vi "USRP Packet Receiver_Global.vi"() -> ()   [LabVIEW 2013]
uses:
  Global 1.vi
  <vilib>/addons/Modulation/niDMT.lvlib
panel:
  in  "16-PSK System Parameters":T1={"Samples per Symbol"=8, "symbol map"=[], "Differential PSK"=enum."disable", "PSK type"=0} {"PSK type" items=["normal", "shifted", "offset"]; "symbol map" format="%.3f"}
  in  "8-PSK System Parameters":T1={"Samples per Symbol"=8, "symbol map"=[], "Differential PSK"=enum."disable", "PSK type"=0} {"PSK type" items=["normal", "shifted", "offset"]; "symbol map" format="%.3f"}
  in  "QPSK System Parameters":T1={"Samples per Symbol"=8, "symbol map"=[], "Differential PSK"=enum."disable", "PSK type"=0} {"PSK type" items=["normal", "shifted", "offset"]; "symbol map" format="%.3f"}
  in  "BPSK System Parameters":T1={"Samples per Symbol"=8, "symbol map"=[], "Differential PSK"=enum."disable", "PSK type"=0} {"PSK type" items=["normal", "shifted", "offset"]; "symbol map" format="%.3f"}
  out "Sync Found":bool
  out "Recovered Message":string
  out "Received Signal (Raw)":dbl[](graph)
  out "Constellation Graph":T2(graph)
  in  "filter parameters":T3={"Alpha"=0.5, "Filter Length"=6, "TX Filter"=enum."Root Raised Cos"} caption="Matching Filter Parameters" {"Alpha" format="%.2f"}
  in  "Modulation type":string(combo)="QPSK"
  in  "Rx IQ Sampling\nRate [s/sec]":dbl=400000.0 format="%#.6p"
  out "Symbol Rate [symbols/sec]":dbl=25000.0 format="%#.6p"
  out "Correct Packets Rx":i16
  in  "Continuous Acquire?":bool
  out "Singal & Noise Power":cluster{"signal_power":dbl, "noise_power":dbl}={"signal_power"=1.4546950663593878e-09, "noise_power"=2.571229598792933e-12}
  out "Cumulative Packets Recovered":i16(graph)
  out "Signal and Noise Power Tracking":cluster{"total_power":dbl, "noise_power":dbl}(graph)={"total_power"=1.4546950663593878e-09, "noise_power"=2.571229598792933e-12}
  in  "PN Sequence Order for Sync":i32=31
  in  "Packet Parameters":T4={"Guard Bits "=30, "Sync Bits"=20, "Message Bits"=128, "Number of Packets \nto Expect"=46}
  in  "synchronization parameters":T5={"expected sync location (symbols)"=-1, "sync sequence"=[], "sync location uncertainty (symbols)"=0, "sync indent (symbols)"=0} {"sync sequence" format="%.2f"}
  in  "stop":bool
  # "Guard\nBand"
  # "Sync\nSeq"
  # "Packet\nNumber"
  # "Pad\nData"
  # "Data"
  # "Packet Receiver"
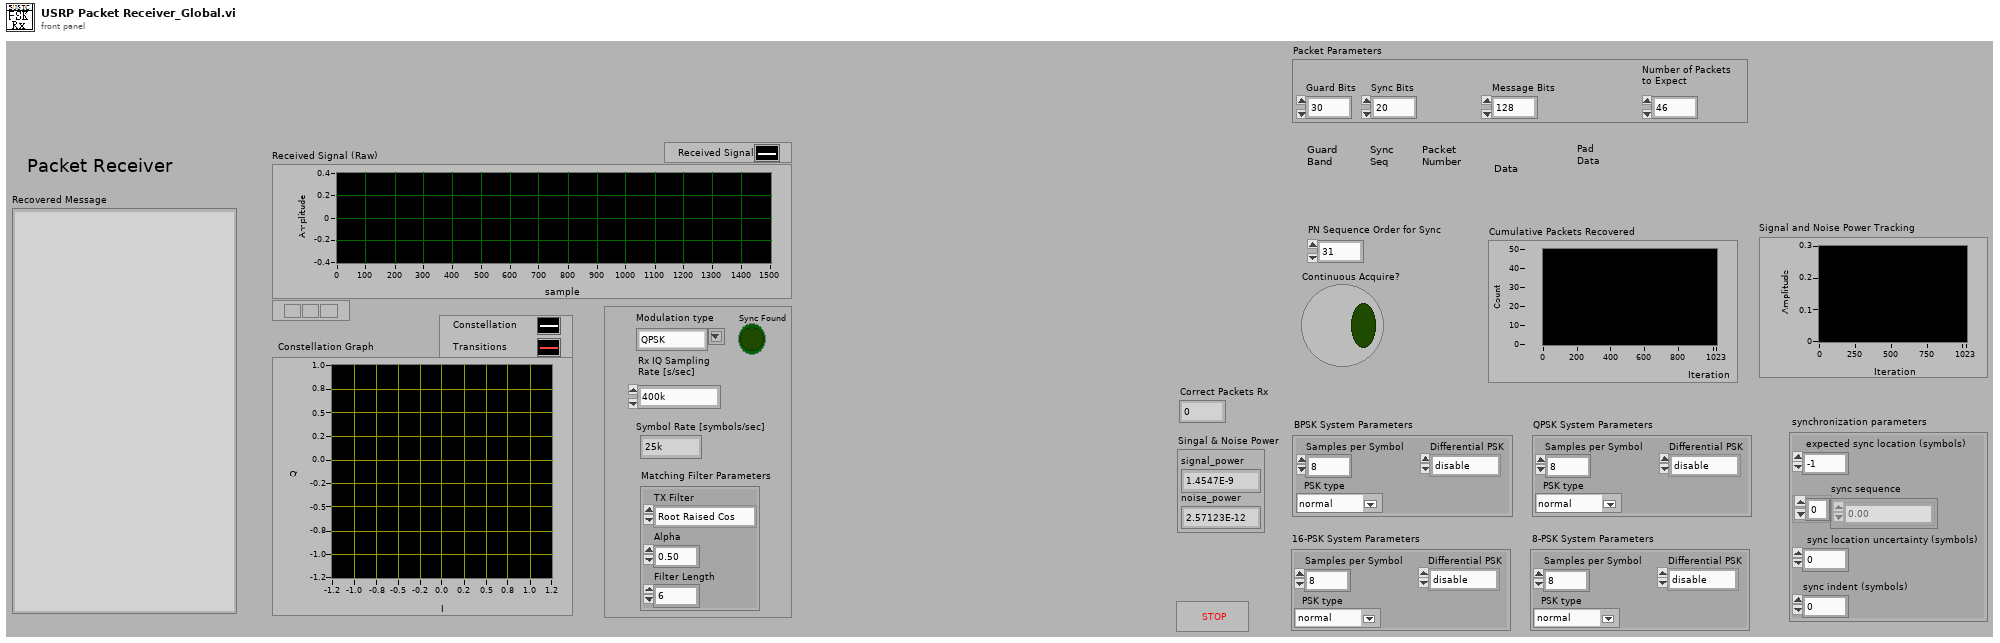
[diagram p1: front panel]
types:
  T1 = cluster{"Samples per Symbol":i32, "symbol map":cdb[], "Differential PSK":enum16{"disable", "enable"}, "PSK type":u16}
  T2 = cluster{"Decimated Array":dbl[], "Decimated Array":dbl[]}[]
  T3 = cluster{"Alpha":dbl, "Filter Length":i32, "TX Filter":enum16{"none", "Raised Cosine", "Root Raised Cos", "Gaussian"}}
  T4 = cluster{"Guard Bits ":i32, "Sync Bits":i32, "Message Bits":i32, "Number of Packets \nto Expect":i32}
  T5 = cluster{"expected sync location (symbols)":i32, "sync sequence":cdb[], "sync location uncertainty (symbols)":i32, "sync indent (symbols)":i32}
  T6 = cluster{"Packet Array":i32[][], "IP Array of Pkt Nums Received  ":bool[]}
  T7 = cluster{"bit stream ":i8[][], "Sync Valid?":bool[], "Decoded Pkt Numbers":u32[], "Enable?":bool}
  T8 = cluster{"packet_arr":cdb[][], "Packets Valid?":bool}
  T9 = cluster{"PSK type":u16, "Samples per Symbol":i32, "Differential PSK":enum16{"disable", "enable"}, "M-PSK (4)":i32}
  T10 = cluster{"PSK system parameters":cluster{"samples per symbol (16)":i32, "symbol map":cdb[], "differential PSK":enum16{"disable", "enable"}, "PSK type":u16}, "pulse shaping filter coefficients":dbl[], "matched filter coefficients":dbl[], "synchronization parameters":cluster{"expected sync location (symbols)":i32, "sync sequence":cdb[], "sync location uncertainty (symbols)":i32, "sync indent (symbols)":i32}, "Sync Bits":i8[]}
  T11 = typedef "niAMT.lvlib/Complex Data Waveform.ctl" = cluster{"t0":dbl, "dt":dbl, "Y":cdb[]}
  T12 = cluster{"constellation":dbl[], "oversampled data":dbl[]}[]
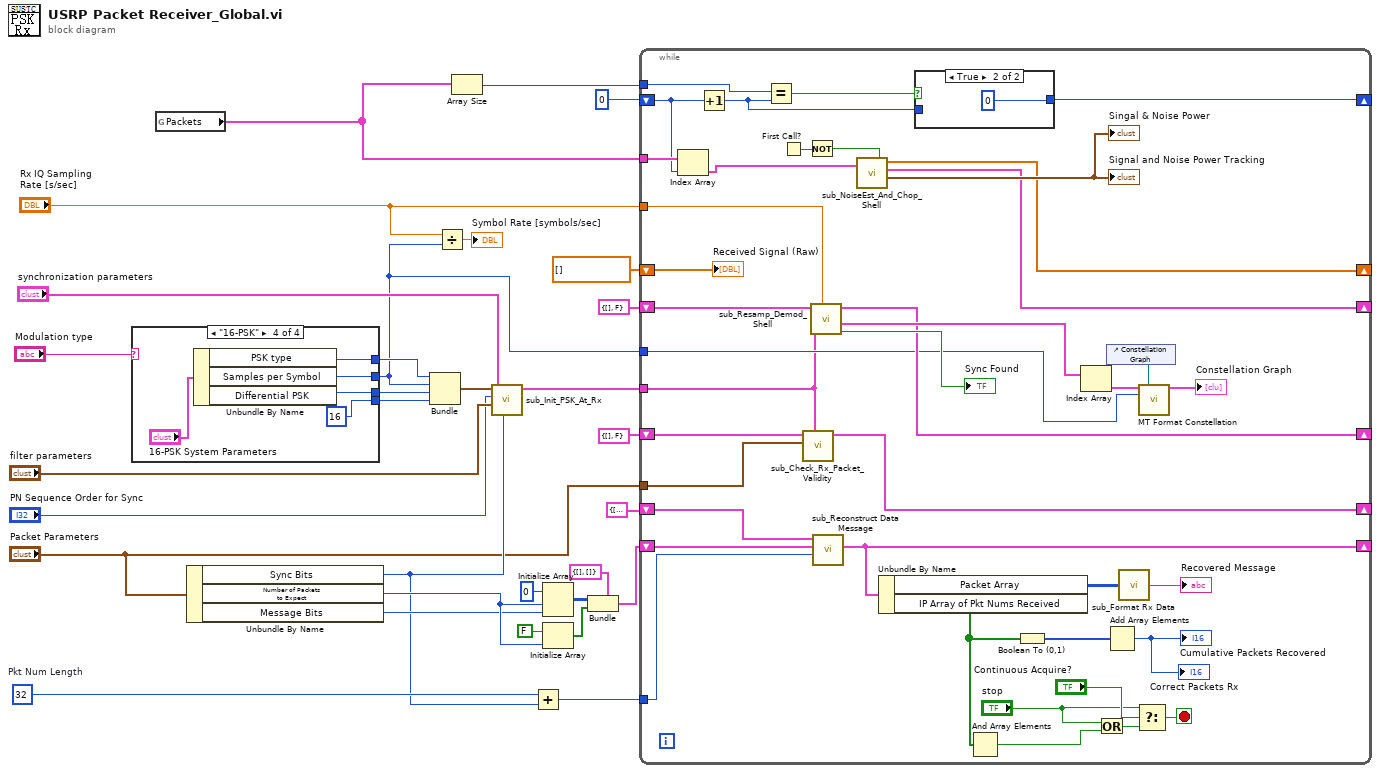
[diagram p0: block diagram]
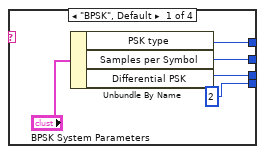
[diagram p3: hidden frame]
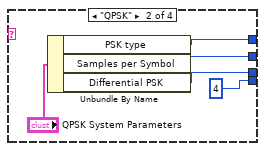
[diagram p4: hidden frame]
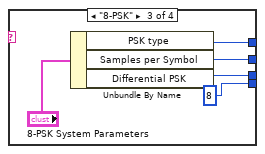
[diagram p5: hidden frame]
diagram:
  w21 = 32  # Pkt Num Length
  n1 = case shown="\"16-PSK\"" "Modulation type" {
    tunnel: [w34 w40 w45 w51] -> w4
    tunnel: [w35 w38 w44 w50] -> w27
    tunnel: [2 ("M-PSK (4)") 4 ("M-PSK (4)") 8 ("M-PSK (4)") 16 ("M-PSK (4)")] -> w26
    tunnel: [w36 w39 w46 w49] -> w28
    frame "BPSK", Default {
      n2 = Unbundle By Name("BPSK System Parameters") -> ("PSK type"=w36:u16, "Samples per Symbol"=w34:i32, "Differential PSK"=w35:enum16{"disable", "enable"})
    }
    frame "QPSK" {
      n3 = Unbundle By Name("QPSK System Parameters") -> ("PSK type"=w39:u16, "Samples per Symbol"=w40:i32, "Differential PSK"=w38:enum16{"disable", "enable"})
    }
    frame "8-PSK" {
      n4 = Unbundle By Name("8-PSK System Parameters") -> ("PSK type"=w46:u16, "Samples per Symbol"=w45:i32, "Differential PSK"=w44:enum16{"disable", "enable"})
    }
    frame "16-PSK" {
      n5 = Unbundle By Name("16-PSK System Parameters") -> ("PSK type"=w49:u16, "Samples per Symbol"=w51:i32, "Differential PSK"=w50:enum16{"disable", "enable"})
    }
  }
  n6 = global read "Global 1.vi" "Packets"() -> (w2:cluster{"t0":dbl, "dt":dbl, "Y":cdb[]}[])
  n7 = Unbundle By Name("Packet Parameters") -> ("Sync Bits"=w12:i32, "Number of Packets \nto Expect"=w20:i32, "Message Bits"=w19:i32)
  n8 = Bundle("PSK type"=w28, "Samples per Symbol"=w4, "Differential PSK"=w27, "M-PSK (4)"=w26) -> (w24:T9)  [unwired: 1 in]
  n9 = Divide(x="Rx IQ Sampling\nRate [s/sec]", y=w4) -> (x/y=→"Symbol Rate [symbols/sec]":dbl)
  n10 = Array Size(array=w2) -> (size(s)=w1:i32)
  n11 = call "sub_Init_PSK_At_Rx.vi"("Sync Bits"=w12, "synchronization parameters"="synchronization parameters", "filter parameters"="filter parameters", "PN sequence order (9)"="PN Sequence Order for Sync", "PSK Parameters"=w24) -> ("PSK Init Parameters"=w23:T10)  [unwired: 5 in, 1 out]
  n12 = Add(x=w21, y=w12) -> (x+y=w29:i32)
  n13 = Initialize Array(0, w20, w19) -> (w14:i32[][])
  n14 = Initialize Array(FALSE, w20) -> (w13:bool[])
  n15 = Bundle(cluster=T6 {"Packet Array"=[], "IP Array of Pkt Nums Received  "=[]} ("Packet Info"), "Packet Array"=w14, "IP Array of Pkt Nums Received"=w13) -> (w9:T6)
  n16 = while {
    tunnel: "Rx IQ Sampling\nRate [s/sec]" -> [w91]
    tunnel: "Packet Parameters" -> [w90]
    tunnel: w29 -> [w68]
    tunnel: w23 -> [w61]
    tunnel: w4 -> [w62]
    shift-right: [w66] -> _
    shift-left: w9 -> [w69]
    shift-right: [w73] -> _
    shift-left: T8 {"packet_arr"=[], "Packets Valid?"=FALSE} -> [w74]
    shift-right: [w71] -> _
    shift-left: cluster{"bit stream":i8[][], "Enable?":bool} {"bit stream"=[], "Enable?"=FALSE} ("Output Bitstream") -> [w72]
    shift-right: [w60] -> _
    shift-left: T7 {"bit stream "=[], "Sync Valid?"=[], "Decoded Pkt Numbers"=[], "Enable?"=FALSE} ("Output Bit Stream") -> [w70]
    shift-right: [w63] -> _
    shift-left: cdb[] [] ("Delay signal (for plotting use only)") -> [w64]
    shift-right: [w53] -> _
    shift-left: 0 -> [w52]
    tunnel: w2 -> [w57]
    tunnel: w1 -> [w55]
    stop <- w86 stop-if-true
    n17 = Index Array(array=w57, index=w52) -> (element=w56:cluster{"t0":dbl, "dt":dbl, "Y":cdb[]})
    n18 = Increment(x=w52) -> (x+1=w54:i32)
    n19 = Equal?(x=w55, y=w54) -> (x = y?=w58:bool)
    n20 = First Call?() -> (First Call?: T/F=w77:bool)
    n21 = call "sub_Check_Rx_Packet_Validity.vi"("PSK Init Parameters"=w61, "Packet Parameters"=w90, "Input Bit Stream"=w72) -> ("Output Bit Stream"=w60:T7)  [unwired: 7 in]
    n22 = Not(x=w77) -> (.not. x?=w76:bool)
    n23 = call "sub_Resamp_Demod_Shell.vi"("Rx IQ Sampling\nRate [s/sec]"=w91, "PSK Init Parameters"=w61, "Input Packets"=w74) -> ("Synch Found?"=→"Sync Found":bool, "recovered complex waveform"=w79:T11[], "Output Bitstream"=w71:cluster{"bit stream":i8[][], "Enable?":bool})  [unwired: 3 in]
    n24 = call "sub_Reconstruct Data Message.vi"("Start Loc of Data"=w68, "Packet Info"=w69, "Input Stream"=w70) -> ("Packet Info out"=w66:T6)  [unwired: 8 in]
    n25 = call "sub_NoiseEst_And_Chop_Shell.vi"("data"=w56, "Enable"=w76) -> ("Singal & Noise Power"=→"Signal and Noise Power Tracking" →"Singal & Noise Power":cluster{"signal_power":dbl, "noise_power":dbl}, "Output Packets"=w73:cluster{"Packets":cdb[][], "Enable?":bool}, "Delay signal (for plotting use only)"=w63:cdb[])  [unwired: 3 in]
    n26 = Unbundle By Name(w66) -> ("Packet Array"=w67:i32[][], "IP Array of Pkt Nums Received"=w65:bool[])
    n27 = case shown="True" w58 {
      tunnel: w54 -> [w92 _]
      tunnel: [w92 0] -> w53
      frame False {
      }
      frame True {
      }
    }
    n28 = And Array Elements(Boolean array=w65) -> (logical AND=w59:bool)
    n29 = Boolean To (0,1)(Boolean=w65) -> (0, 1=w89:i16[])
    n30 = Index Array(array=w79) -> (element=w78:T11)  [unwired: 1 in]
    n31 = Or(x="stop", y=w59) -> (x .or. y?=w87:bool)
    n32 = control-ref of="Constellation Graph"() -> (w81:refnum<vi>)
    n33 = Add Array Elements(numeric array=w89) -> (sum=→"Correct Packets Rx" →"Cumulative Packets Recovered":i16)
    n34 = call "sub_Format Rx Data.vi"("Output Packet Array"=w67) -> ("Received Message"=→"Recovered Message":string)
    n35 = Select(t="stop", s="Continuous Acquire?", f=w87) -> (s? t:f=w86:bool)
    n36 = call <vilib>:"MT Format Constellation.vi"("waveform"=w78, "constellation reference"=w81, "samples per symbol"=w62) -> ("constellation graph"=→"Constellation Graph":T12)  [unwired: 2 in, 10 out]
    "Received Signal (Raw)" <- w64
  }
